vi "Demo_DatabaseTest.vi"() -> ()   [LabVIEW 2016]
uses:
  database/database.lvlib
panel:
  in  "错误输入 16":errorcluster caption="错误输入"
  in  "TestId":string
  in  "dataLabel":string
  in  "content":string
  in  "msgid":dbl
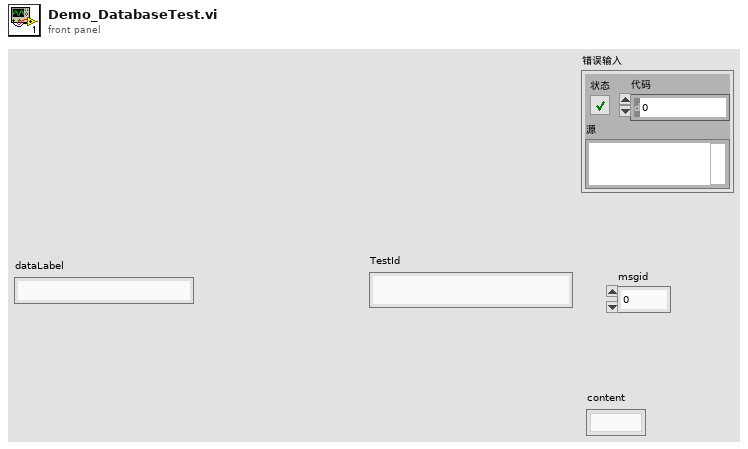
[diagram p1: front panel]
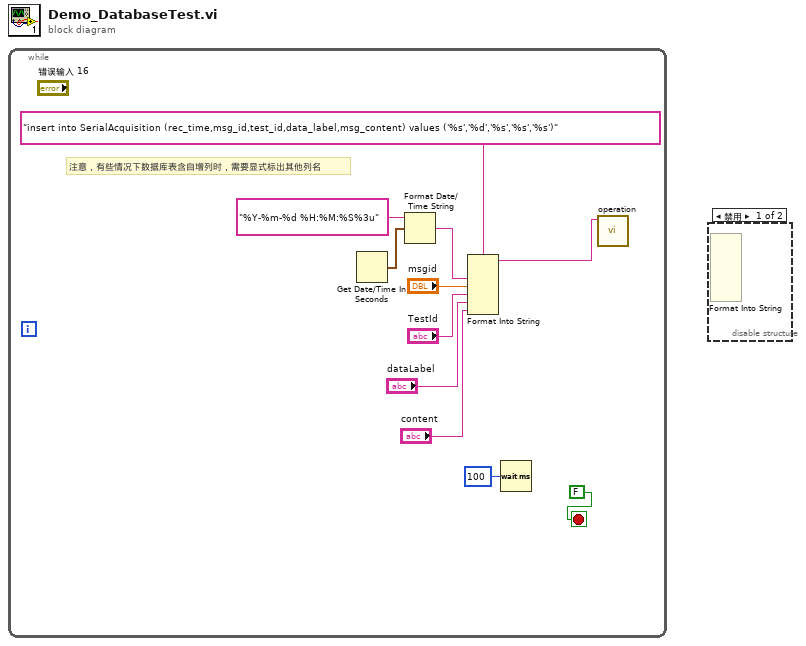
[diagram p0: block diagram]
diagram:
  n1 = while {
    stop <- FALSE stop-if-true
    # "注意，有些情况下数据库表含自增列时，需要显式标出其他列名"
    n2 = Get Date/Time In Seconds() -> (seconds since 1Jan1904=w9:timestamp)
    n3 = Format Date/Time String ("格式化日期/时间字符串")(time format string (%c)="%Y-%m-%d %H:%M:%S%3u" ("时间格式字符串(%c)"), seconds (now)=w9) -> (date/time string=w6:string)  [unwired: 1 in]
    n4 = Format Into String(format string="insert into SerialAcquisition (rec_time,msg_id,test_id,data_label,msg_content) values ('%s','%d','%s','%s','%s')" ("格式字符串"), w6, "msgid", "TestId", "dataLabel", "content") -> (resulting string=w1:string)  [unwired: 2 in, 1 out]
    n5 = Wait (ms)(milliseconds to wait=u32 100) -> ()  [unwired: 1 out]
    n6 = call "operation.vi"("Command Text"=w1) -> ()  [unwired: 9 in, 1 out]
  }
  n7 = disable-structure shown="禁用" {
    frame Disabled {
      n8 = Format Into String() -> ()  [unwired: 9 in, 2 out]
    }
    frame Enabled {
    }
  }
